vi "Dummy.vi"   [LabVIEW 2014]
uses:
  <vilib>/DAQmx/write.llb/DAQmx Write (Digital Bool 1Line 1Point).vi
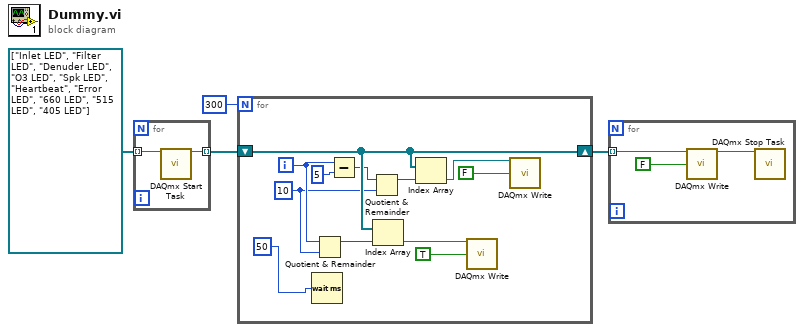
[diagram p0: block diagram]
diagram:
  n1 = for {
    tunnel: refnum<k21>[] ["Inlet LED", "Filter LED", "Denuder LED", "O3 LED", "Spk LED", "Heartbeat", "Error LED", "660 LED", "515 LED", "405 LED"] -> [w6] mode=indexing
    tunnel: [w5] -> w3 mode=indexing
    n2 = call <vilib>:"DAQmx Start Task.vi"("task/channels in"=w6) -> ("task out"=w5:refnum<k21>)  [unwired: 13 in, 1 out]
  }
  n3 = for {
    N: 300 -> [_]
    shift-right: [w13] -> w2
    shift-left: w3 -> [w13]
    i -> [w16]
    w11 = 10 ("y")
    n4 = Wait (ms)(milliseconds to wait=u32 50) -> ()  [unwired: 1 out]
    n5 = Quotient & Remainder(x=w16, y=w11) -> (x-y*floor(x/y)=w15:i32)  [unwired: 1 out]
    n6 = Subtract(x=w16, y=5) -> (x-y=w12:i32)
    n7 = Quotient & Remainder(x=w12, y=w11) -> (x-y*floor(x/y)=w10:i32)  [unwired: 1 out]
    n8 = Index Array(array=w13, index=w15) -> (element=w14:refnum<k21>)
    n9 = Index Array(array=w13, index=w10) -> (element=w9:refnum<k21>)
    n10 = call-poly <vilib>:"DAQmx Write.vi"("task/channels in"=w14, "data"=TRUE) -> ()  [unwired: 11 in, 3 out]
    n11 = call-poly <vilib>:"DAQmx Write.vi"("task/channels in"=w9, "data"=FALSE) -> ()  [unwired: 11 in, 3 out]
  }
  n12 = for {
    tunnel: w2 -> [w20] mode=indexing
    n13 = call-poly <vilib>:"DAQmx Write.vi"("task/channels in"=w20, "data"=FALSE) -> ("task out"=w19:refnum<k21>)  [unwired: 11 in, 2 out]
    n14 = call <vilib>:"DAQmx Stop Task.vi"("task/channels in"=w19) -> ()  [unwired: 13 in, 2 out]
  }
